vi "GetMeasurementResult.vi"(8 "error in (no error)":errorcluster, 11 "MeasuringDevice in":refnum<class "MeasuringDevice.lvclass">) -> (0 "error out":errorcluster, 2 "Result":variant, 3 "MeasuringDevice out":refnum<class "MeasuringDevice.lvclass">)   [LabVIEW 2017, in "MeasuringDevice.lvclass"]
uses:
  MeasuringDevice.lvclass
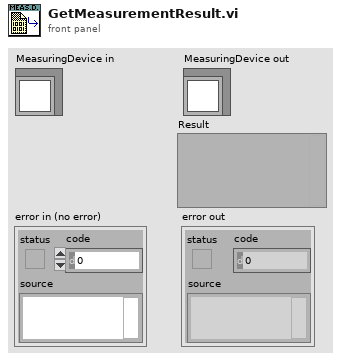
[diagram p1: front panel]
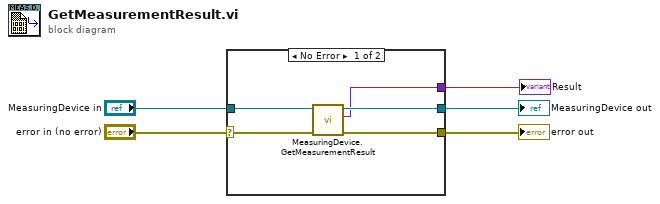
[diagram p0: block diagram]
diagram:
  n1 = case shown="No Error" "error in (no error)" {
    selector: "error in (no error)" -> [w9 w12]
    tunnel: [w8 w12] -> w4
    tunnel: [w7 w11] -> w2
    tunnel: "MeasuringDevice in" -> [w10 w11]
    tunnel: [w6 _] -> w1
    frame No Error {
      n2 = call-dynamic "MeasuringDevice.GetMeasurementResult.vi"("error in (no error)"=w9, "MeasuringDevice"=w10) -> ("error out"=w8:errorcluster, "Result"=w6:variant, "MeasuringDevice out"=w7:refnum<class "MeasuringDevice.lvclass">)  [unwired: 7 in]
    }
    frame Error {
    }
  }
  "error out" <- w4
  "MeasuringDevice out" <- w2
  "Result" <- w1
